vi "Gas Heater Test.vi"(8 "error in":errorcluster) -> (0 "error out":errorcluster)   [LabVIEW 2014]
uses:
  CAN Communication/Peltier/Typedefs/Peltier Temperature Sensors.ctl
  CAN Communication/Peltier/Peltier.lvclass
  CAN Communication/PAS/PAS.lvclass
panel:
  in  "Stop":bool
  out "TS5":dbl
  out "Timeout":i32
  out "Error":errorcluster
  # "Gas Heater Test"
  # "This test performs functionality\ntesting on the Gas Heater.\n\nPlease standby while the test is\nin progress..."
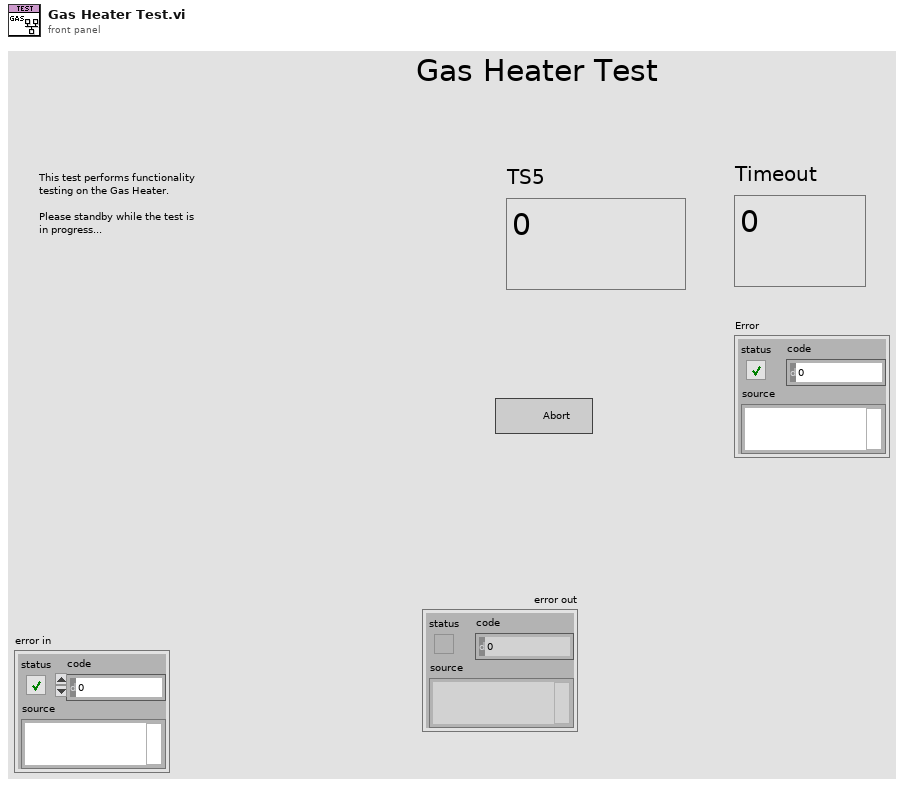
[diagram p1: front panel]
types:
  T1 = typedef "Peltier.lvclass/Peltier Temperature Sensors.ctl" = u16
  T2 = typedef "PAS.lvclass/Session Handle.ctl" = refnum<data-value>
  T3 = typedef "Peltier.lvclass/Session Handle.ctl" = refnum<data-value>
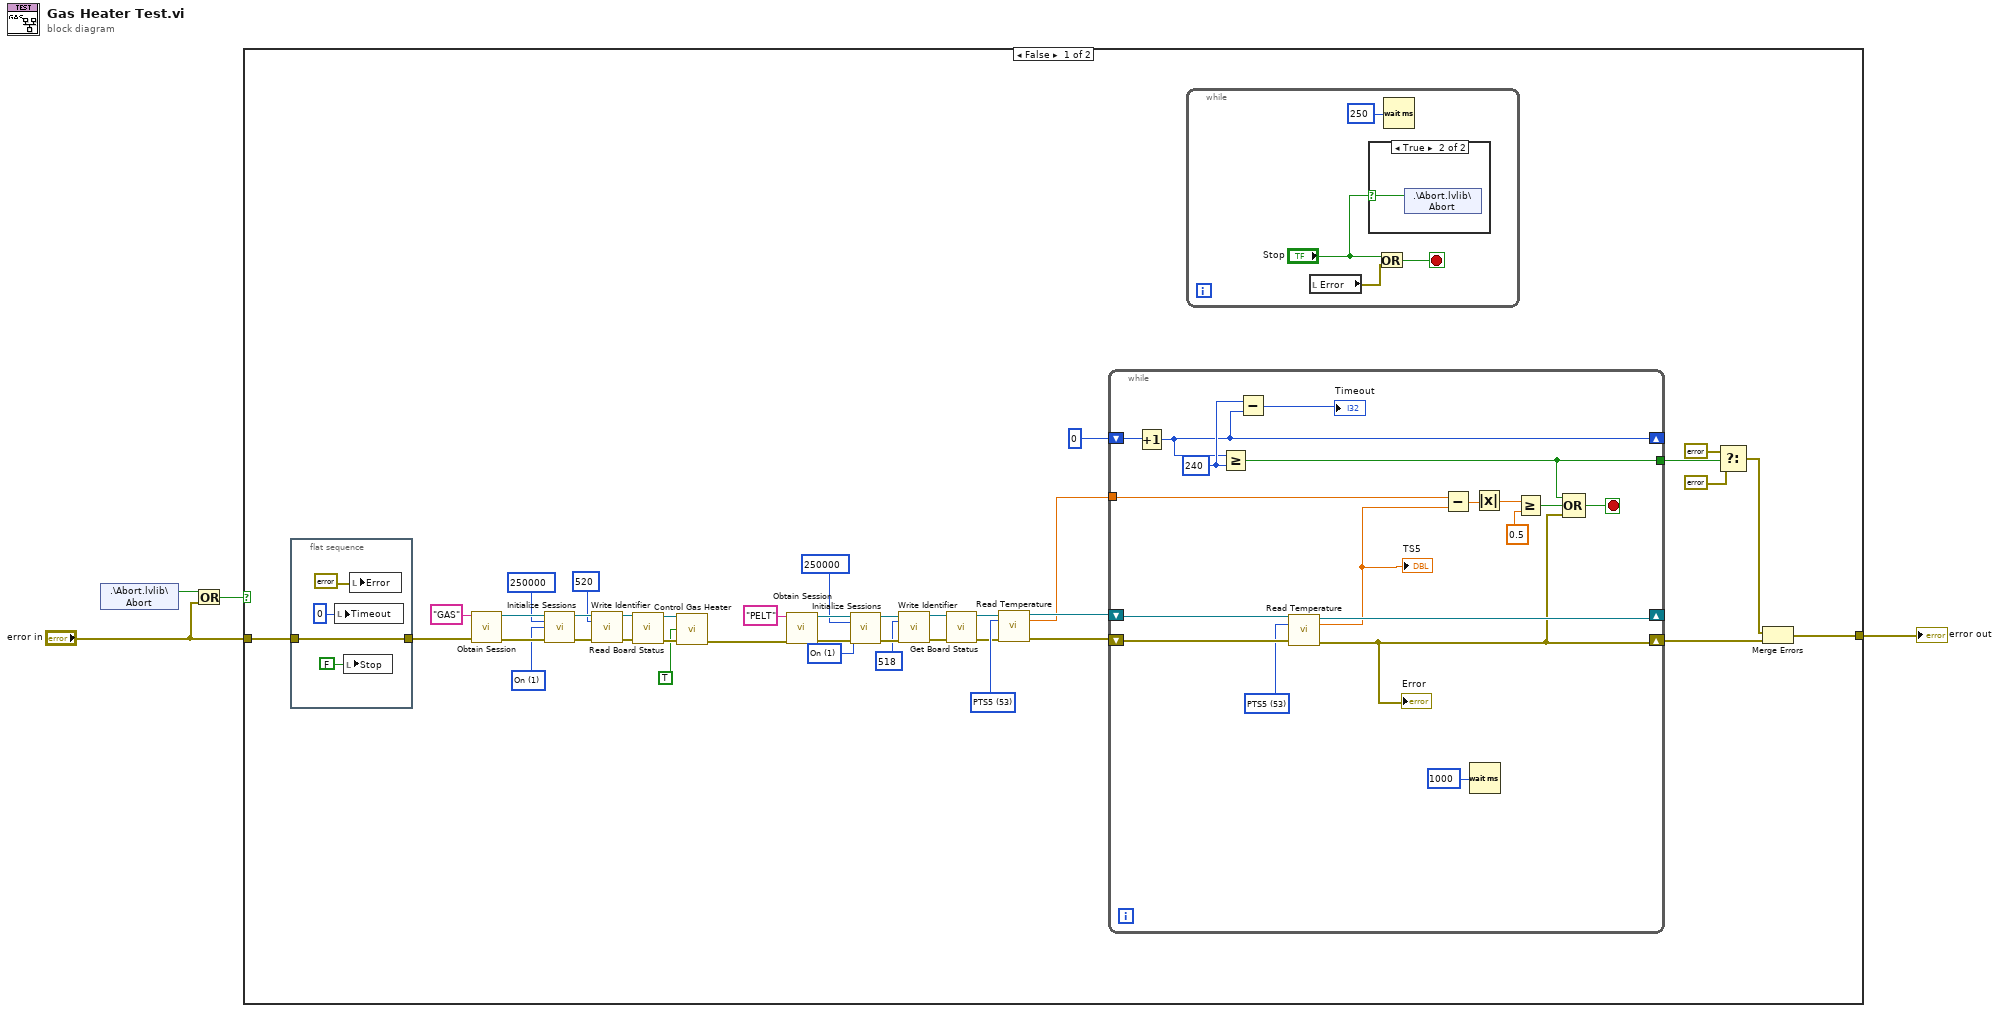
[diagram p0: block diagram]
diagram:
  n1 = shared-variable ".\\Abort.lvlib\\Abort"() -> (w3:bool)  [unwired: 1 in, 1 out]
  n2 = Or(x=w3, y="error in") -> (x .or. y?=w1:bool)
  n3 = case shown="False" w1 {
    tunnel: [w23 w71] -> w4
    tunnel: "error in" -> [w6 w71]
    frame False {
      w17 = u32 1 items=["Off", "On"] ("Termination")
      w31 = T1 53 items=["PTS1"=49, "PTS2"=50, "PTS3"=51, "PTS4"=52, "PTS5"=53, "PTS6"=54] ("Pelt Temp Sensors")
      w39 = u32 1 items=["Off", "On"] ("Termination")
      n4 = flat-sequence {
        tunnel: [w47] -> w5
        tunnel: w6 -> [w47]
        frame #0 {
          n5 = local write "Timeout"(0 ("Timeout")) -> ()
          n6 = local write "Stop"(FALSE ("Stop")) -> ()
          n7 = local write "Error"(errorcluster {"status"=FALSE, "code"=0, "source"=""} ("Peltier Errors")) -> ()
        }
      }
      n8 = call "Obtain Session.vi"("Session  Name ()"="GAS", "error in (no error)"=w5) -> ("Session Handle"=w21:T2, "error out"=w20:errorcluster)  [unwired: 12 in]
      n9 = call "Initialize Sessions.vi"("Session Handle in"=w21, "Baud Rate"=u32 250000, "Termination"=w17, "error in (no error)"=w20) -> ("Session Handle Out"=w16:T2, "error out"=w15:errorcluster)  [unwired: 10 in]
      n10 = call "Write Identifier.vi"("Session Handle in"=w16, "identifier"=u16 520, "error in (no error)"=w15) -> ("Session Handle out"=w13:T2, "error out"=w12:errorcluster)  [unwired: 11 in]
      n11 = call "Read Board Status.vi"("Session Handle in"=w13, "error in (no error)"=w12) -> ("Session Handle out"=w11:T2, "error out"=w10:errorcluster)  [unwired: 11 in, 1 out]
      n12 = call "Control Gas Heater.vi"("Session Handle in"=w11, "On?"=TRUE, "error in (no error)"=w10) -> ("error out"=w9:errorcluster)  [unwired: 10 in, 2 out]
      n13 = call "Obtain Session.vi"("Session  Name ()"="PELT", "error in (no error)"=w9) -> ("Session Handle"=w42:T3, "error out"=w41:errorcluster)  [unwired: 12 in]
      n14 = call "Initialize Sessions.vi"("Session Handle"=w42, "Baud Rate"=u32 250000, "Termination"=w39, "error in (no error)"=w41) -> ("Session Handle Out"=w38:T3, "error out"=w37:errorcluster)  [unwired: 10 in]
      n15 = call "Write Identifier.vi"("Session Handle In"=w38, "identifier"=u16 518, "error in (no error)"=w37) -> ("Session Handle Out"=w35:T3, "error out"=w34:errorcluster)  [unwired: 11 in]
      n16 = call "Get Board Status.vi"("Session Handle"=w35, "error in (no error)"=w34) -> ("Session Handle Out"=w7:T3, "error out"=w22:errorcluster)  [unwired: 11 in, 1 out]
      n17 = call "Read Temperature.vi"("Session Handle"=w7, "Pelt Temp Sensors"=w31, "error in (no error)"=w22) -> ("Session Handle Out"=w32:T3, "Temperature"=w30:dbl, "error out"=w33:errorcluster)  [unwired: 10 in]
      n18 = while {
        shift-right: [w69] -> _
        shift-left: w32 -> [w56]
        shift-right: [w63] -> w24
        shift-left: w33 -> [w55]
        tunnel: w30 -> [w68]
        shift-right: [w58] -> _
        shift-left: 0 -> [w61]
        tunnel: [w60] -> w25
        stop <- w62 stop-if-true
        w54 = T1 53 items=["PTS1"=49, "PTS2"=50, "PTS3"=51, "PTS4"=52, "PTS5"=53, "PTS6"=54] ("Pelt Temp Sensors")
        w59 = 240 ("y")
        n19 = Increment(x=w61) -> (x+1=w58:i32)
        n20 = Greater Or Equal?(x=w58, y=w59) -> (x >= y?=w60:bool)
        n21 = Subtract(x=w59, y=w58) -> (x-y=→"Timeout":i32)
        n22 = call "Read Temperature.vi"("Session Handle"=w56, "Pelt Temp Sensors"=w54, "error in (no error)"=w55) -> ("Session Handle Out"=w69:T3, "Temperature"=w53:dbl, "error out"=w63:errorcluster)  [unwired: 10 in]
        "Error" <- w63
        "TS5" <- w53
        n23 = Subtract(x=w68, y=w53) -> (x-y=w67:dbl)
        n24 = Wait (ms)(milliseconds to wait=u32 1000) -> ()  [unwired: 1 out]
        n25 = Absolute Value(x=w67) -> (abs(x)=w66:dbl)
        n26 = Greater Or Equal?(x=w66, y=0.5) -> (x >= y?=w64:bool)
        n27 = Compound Arithmetic op=OR(w60, w64, w63) -> (w62:bool)
      }
      n28 = while {
        stop <- w50 stop-if-true
        n29 = local read "Error"() -> (w48:errorcluster)
        n30 = case shown="True" "Stop" {
          selector: "Stop" -> [_ w52]
          frame False {
          }
          frame True {
            n31 = shared-variable ".\\Abort.lvlib\\Abort"(w52) -> ()  [unwired: 1 in, 1 out]
          }
        }
        n32 = Or(x="Stop", y=w48) -> (x .or. y?=w50:bool)
        n33 = Wait (ms)(milliseconds to wait=u32 250) -> ()  [unwired: 1 out]
      }
      n34 = Select(t=errorcluster {"status"=TRUE, "code"=9002, "source"="Timeout Error. Gas Heater failed to impact Peltier Temperature Sensor."} ("error out"), s=w25, f=errorcluster {"status"=FALSE, "code"=0, "source"=""} ("error out")) -> (s? t:f=w26:errorcluster)
      n35 = Merge Errors(w26, w24) -> (w23:errorcluster)
    }
    frame True {
    }
  }
  "error out" <- w4
